vi "Check Status.vi"(8 "Error In":errorcluster, 10 "Status":i32, 11 "libssh2lv Shared Library In":path=path "") -> (0 "Error Out":errorcluster, 3 "libssh2lv Shared Library Out":path)   [LabVIEW 2018, in "Toolkit.lvlib"]
doc: "Determines the result of the function call from the libssh2lv shared library and converts failures to an error."
uses:
  Toolkit.lvlib
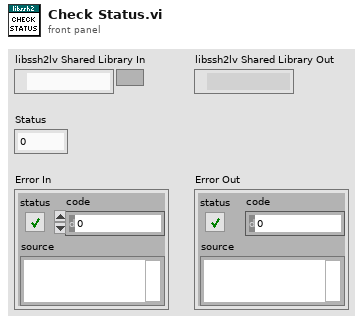
[diagram p1: front panel]
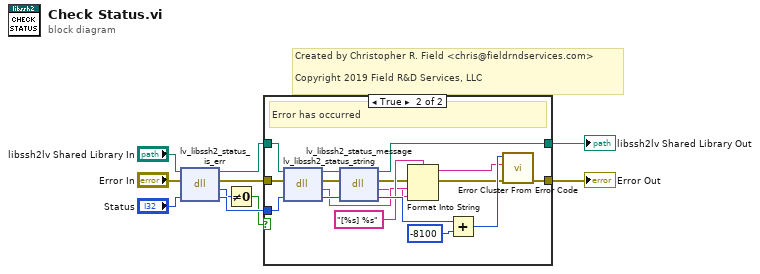
[diagram p0: block diagram]
diagram:
  # "Created by Christopher R. Field <chris@fieldrndservices.com>\n\nCopyright 2019 Field R&D Services, LLC"
  n1 = dll-call lib="D:/Users/cfield/Code/Field R&D Services/SSH/LV-LIBSSH2/LabVIEW/trunk/src/Toolkit/Support/lv-libssh2.*" fn="lv_libssh2_status_is_err"(path in="libssh2lv Shared Library In", error in="Error In", "status"="Status") -> (path out=w9:path, error out=w7:errorcluster, "bool"=w2:i32, "status"=w5:i32)  [unwired: 1 in]
  n2 = Not Equal To 0?(x=w2) -> (x != 0?=w1:bool)
  n3 = case shown="True" w1 {
    tunnel: w9 -> [w12 w26]
    tunnel: w7 -> [w11 w25]
    tunnel: w5 -> [_ w24]
    tunnel: [w12 w23] -> w4
    tunnel: [w11 w20] -> w3
    frame False {
      # "No error"
    }
    frame True {
      # "Error has occurred"
      n4 = dll-call lib="D:/Users/cfield/Code/Field R&D Services/SSH/LV-LIBSSH2/LabVIEW/trunk/src/Toolkit/Support/lv-libssh2.*" fn="lv_libssh2_status_string"(path in=w26, error in=w25, "status"=w24) -> (path out=w27:path, error out=w28:errorcluster, "string"=w14:string, "status"=w29:i32)  [unwired: 1 in]
      n5 = dll-call lib="D:/Users/cfield/Code/Field R&D Services/SSH/LV-LIBSSH2/LabVIEW/trunk/src/Toolkit/Support/lv-libssh2.*" fn="lv_libssh2_status_message"(path in=w27, error in=w28, "status"=w29) -> (path out=w23:path, error out=w17:errorcluster, "message"=w13:string, "status"=w22:i32)  [unwired: 1 in]
      n6 = Format Into String(format string="[%s] %s", error in=w17, w14, w13) -> (resulting string=w15:string, error out=w16:errorcluster)  [unwired: 1 in]
      n7 = Add(x=w22, y=-8100) -> (x+y=w19:i32)
      n8 = call <vilib>:"Error Cluster From Error Code.vi"("error in (no error)"=w16, "error message (\"\")"=w15, "error code (0)"=w19) -> ("error out"=w20:errorcluster)  [unwired: 6 in]
    }
  }
  "libssh2lv Shared Library Out" <- w4
  "Error Out" <- w3
